vi "CacluateSheet.vi"(8 "error in (no error)":errorcluster, 10 "Name":string, 11 "ExcelFile in":refnum<class "PortableExcelFileManipulationOXML.lvclass">) -> (0 "error out":errorcluster, 3 "ExcelFile out":refnum<class "PortableExcelFileManipulationOXML.lvclass">)   [LabVIEW 2019, in "PortableExcelFileManipulationOXML.lvclass"]
doc: "Adds a worksheet to the This excel File by name."
uses:
  PortableExcelFileManipulationOXML.lvclass
  PortableExcelFileManipulationOXML.lvclass/PortableExcelFileManipulationOXML.ctl
  H:/LV projects/ExpressionEvaluator/Excel/ExcelManipulation.dll
  ExcelManipulation.dll
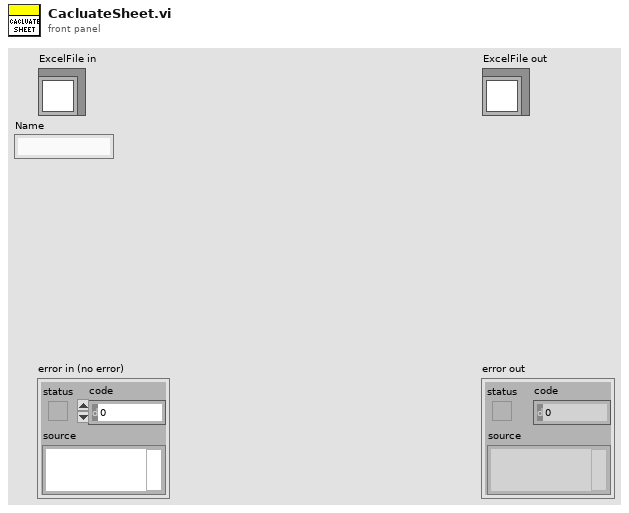
[diagram p1: front panel]
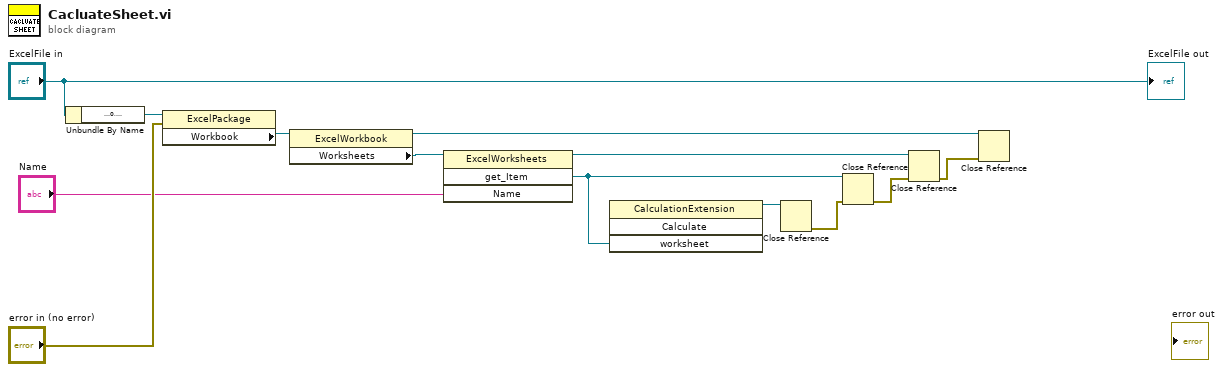
[diagram p0: block diagram]
diagram:
  n1 = Unbundle By Name("ExcelFile in") -> ("ExcelOpen"=w12:refnum<k24>)
  n2 = property class="ExcelPackage"(reference=w12, error in="error in (no error)") -> ("Workbook"=w11:refnum<k24>)  [unwired: 2 out]
  n3 = property class="ExcelWorkbook"(reference=w11) -> (reference out=w1:refnum<k24>, "Worksheets"=w9:refnum<k24>)  [unwired: 1 in, 1 out]
  n4 = invoke class="ExcelWorksheets" method="get_Item"(reference=w9, "Name"="Name") -> (reference out=w3:refnum<k24>, "get_Item"=w6:refnum<k24>)  [unwired: 2 in, 2 out]
  n5 = invoke class="CalculationExtension" method="Calculate"("worksheet"=w6) -> (reference out=w7:refnum<k24>)  [unwired: 3 in, 3 out]
  n6 = Close Reference(reference=w7) -> (error out=w5:errorcluster)  [unwired: 1 in]
  n7 = Close Reference(reference=w6, error in (no error)=w5) -> (error out=w4:errorcluster)
  n8 = Close Reference(reference=w3, error in (no error)=w4) -> (error out=w2:errorcluster)
  n9 = Close Reference(reference=w1, error in (no error)=w2) -> ()  [unwired: 1 out]
  "ExcelFile out" <- "ExcelFile in"
